vi "Set Device User ID.vi"(8 "Error In":errorcluster, 10 "Device User ID":u16, 11 "LINX Resource":T1) -> (0 "Error Out":errorcluster, 3 "LINX Resource":T1)   [LabVIEW 2013, in "LVH-LINX.lvlib"]
uses:
  <vilib>/LabVIEW Hacker/LINX/LVH-LINX.lvlib
  <vilib>/LabVIEW Hacker/LINX/Private/Type Defs/LINX Ref.ctl
  <vilib>/LabVIEW Hacker/LINX/Private/Type Defs/Platform.ctl
  <vilib>/LabVIEW Hacker/LINX/Private/Type Defs/Interface.ctl
  <vilib>/LabVIEW Hacker/LINX/Private/Device/Type Defs/LINX Device Config.ctl
  <vilib>/LabVIEW Hacker/LINX/Private/Device/Type Defs/TCP Config.ctl
  <vilib>/LabVIEW Hacker/LINX/Private/Type Defs/Device Family.ctl
  <vilib>/LabVIEW Hacker/LINX/Private/Type Defs/Error Type.ctl
  <vilib>/LabVIEW Hacker/LINX/Private/Device/Device.lvlib
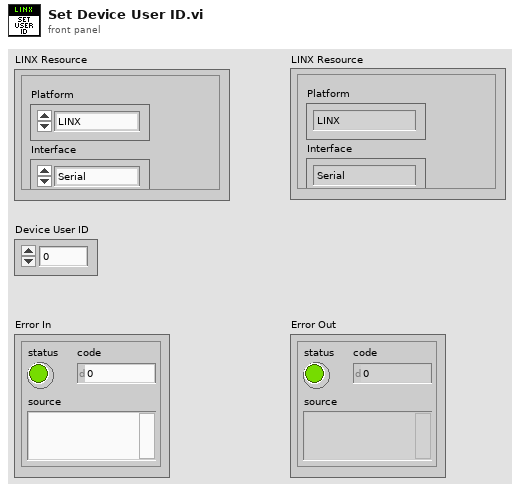
[diagram p1: front panel]
types:
  T1 = typedef "LVH-LINX.lvlib/LINX Ref.ctl" = cluster{"Platform":T2, "Interface":T3, "LINX Device Config":T4}
  T2 = typedef "LVH-LINX.lvlib/Platform.ctl" = enum16{"LINX", "myRIO"}
  T3 = typedef "LVH-LINX.lvlib/Interface.ctl" = enum16{"Serial", "TCP"}
  T4 = typedef "LVH-LINX.lvlib/Device.lvlib/LINX Device Config.ctl" = cluster{"Interface":T3, "COM Port":refnum<visa-resource-name>, "TCP Configuration":T5, "Device Family":T6, "Device ID":u8, "Device Name":string, "TCP Ref":refnum<k5>}
  T5 = typedef "LVH-LINX.lvlib/Device.lvlib/TCP Config.ctl" = cluster{"IP Address":string, "Port":u16}
  T6 = typedef "LVH-LINX.lvlib/Device Family.ctl" = enum8{"National Instruments", "Digilent", "Arduino"}
  T7 = typedef "LVH-LINX.lvlib/Error Type.ctl" = enum16{"Unknown", "Timeout", "Corrupt Return Packet", "Unable To Connect", "Command Not Supported", "Channel DNE", "Invalid COM Config"}
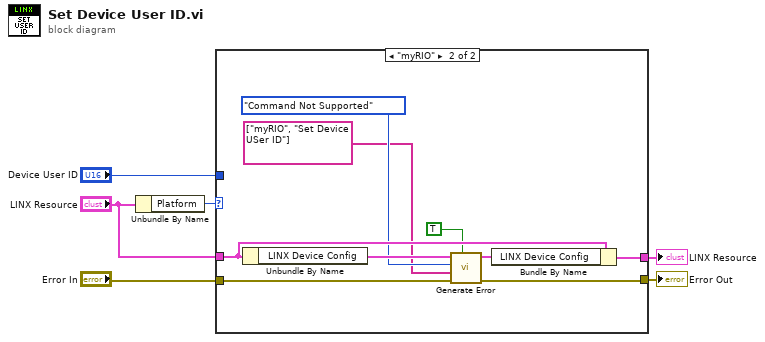
[diagram p0: block diagram]
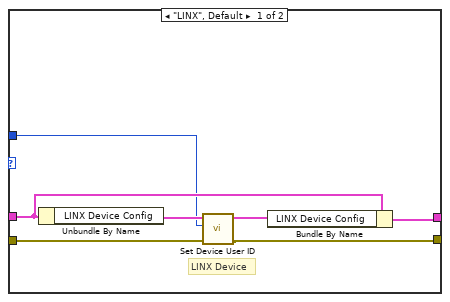
[diagram p2: hidden frame]
diagram:
  n1 = Unbundle By Name("LINX Resource") -> ("Platform"=w6:T2)
  n2 = case shown="\"myRIO\"" w6 {
    tunnel: [w12 w18] -> w5
    tunnel: [w13 w17] -> w1
    tunnel: "Error In" -> [w11 w19]
    tunnel: "LINX Resource" -> [w8 w22]
    tunnel: "Device User ID" -> [w7 _]
    frame "LINX", Default {
      # "LINX Device"
      n3 = Unbundle By Name(w8) -> ("LINX Device Config"=w10:T4)
      n4 = call <vilib>:"Set Device User ID.vi"("Error In"=w11, "Device User ID"=w7, "LINX Device Config"=w10) -> ("Error Out"=w12:errorcluster, "LINX Device Config"=w9:T4)  [unwired: 7 in]
      n5 = Bundle By Name(cluster=w8, "LINX Device Config"=w9) -> (w13:T1)
    }
    frame "myRIO" {
      n6 = Unbundle By Name(w22) -> ("LINX Device Config"=w21:T4)
      n7 = call <vilib>:"Generate Error.vi"("Is Warning? (False)"=TRUE, "Error In"=w19, "Arguments"=string[] ["myRIO", "Set Device USer ID"], "Error Type"=Error_Type."Command Not Supported", "LINX Device Config"=w21) -> ("Error Out"=w18:errorcluster, "LINX Device Config"=w20:T4)  [unwired: 5 in]
      n8 = Bundle By Name(cluster=w22, "LINX Device Config"=w20) -> (w17:T1)
    }
  }
  "Error Out" <- w5
  "LINX Resource" <- w1
